vi "LockinEngine.Test.vi"(8 "error in (no error)":errorcluster, 11 "LockinDAQ in":refnum<class "LockinDAQ.lvclass">) -> (0 "error out":errorcluster, 3 "LockinDAQ out":refnum<class "LockinDAQ.lvclass">)   [LabVIEW 2016, in "LockinDAQ.lvclass"]
uses:
  LockinDAQ.lvclass
  Typedefs/Sampling.ctl
  <vilib>/Analysis/NI_AALBase.lvlib
  <vilib>/Analysis/baseanly.llb/Mean (DBL).vi
  Typedefs/AO_Amp-array.ctl
  Typedefs/AO_DC-array.ctl
  Typedefs/AO_phi-array.ctl
  Typedefs/Function-enum.ctl
  Typedefs/Function-array.ctl
  Typedefs/AO_f-array.ctl
  Typedefs/AO-cluster.ctl
  Typedefs/REF_f-array.ctl
  Typedefs/REF_phi-array.ctl
  Typedefs/REF-cluster.ctl
panel:
  out "Waveform Chart 2":u32(graph)
  out "Average time for each method (ms)":dbl[](array[numeric])
  in  "order":i32=2
  in  "TC (s)":dbl=0.3
  in  "Channels: Lockin":T1={"REF f (Hz)"=[13.0], "REF phi (°)"=[0.0]} {"REF phi (°)" format="%#_3g"}
  out "Waveform Chart":dbl[][](graph)
  in  "AO Chanels":T4={"AO Amp (V)"=[0.01], "AO DC (V)"=[0.0], "AO f (Hz)"=[13.0], "AO Phase (°)"=[0.0], "Function"=[enum."Sine"], "I+"=[], "Sweeping"=[FALSE]} {"AO f (Hz)" min=0.001 max=10000.0; "AO DC (V)" format="%.3p"; "AO Amp (V)" format="%.3p"}
  # "1"
  # "2"
  # "3"
  # "4"
  # "5"
  # "6"
  # "7"
  # "8"
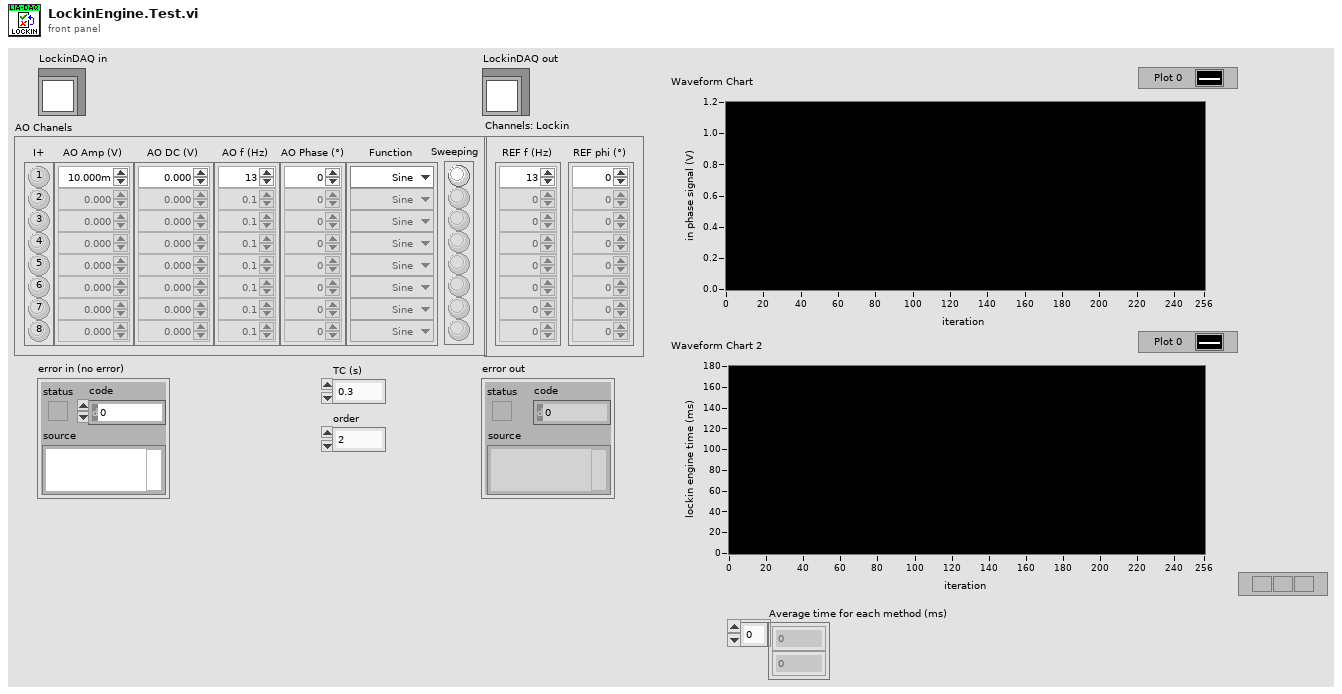
[diagram p1: front panel]
types:
  T1 = typedef "LockinDAQ.lvclass/REF-cluster.ctl" = cluster{"REF f (Hz)":T2, "REF phi (°)":T3}
  T2 = typedef "LockinDAQ.lvclass/REF_f-array.ctl" = dbl[]
  T3 = typedef "LockinDAQ.lvclass/REF_phi-array.ctl" = dbl[]
  T4 = typedef "LockinDAQ.lvclass/AO-cluster.ctl" = cluster{"AO Amp (V)":T5, "AO DC (V)":T6, "AO f (Hz)":T7, "AO Phase (°)":T8, "Function":T9, "I+":bool[], "Sweeping":bool[]}
  T5 = typedef "LockinDAQ.lvclass/AO_Amp-array.ctl" = dbl[]
  T6 = typedef "LockinDAQ.lvclass/AO_DC-array.ctl" = dbl[]
  T7 = typedef "LockinDAQ.lvclass/AO_f-array.ctl" = dbl[]
  T8 = typedef "LockinDAQ.lvclass/AO_phi-array.ctl" = dbl[]
  T9 = typedef "LockinDAQ.lvclass/Function-array.ctl" = T10[]
  T10 = typedef "LockinDAQ.lvclass/Function-enum.ctl" = enum16{"Sine", "Triangle", "Square", "Sawtooth"}
  T11 = enum16{"method 1", "method 2", "method 3", "method 4", "method 5"}[]
  T12 = typedef "LockinDAQ.lvclass/Sampling.ctl" = cluster{"Fs":dbl, "#s":i32}
  T13 = typedef "LockinDAQ.lvclass/Results--Cluster.ctl" = cluster{"Time Stamp":timestamp, "Results":dbl[][]}
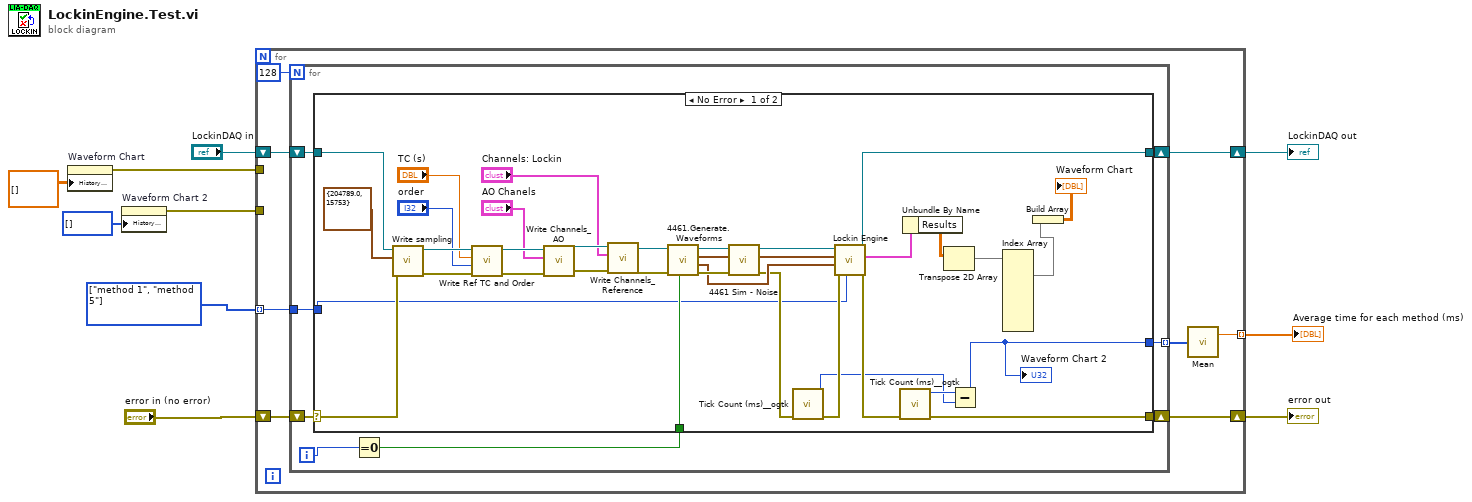
[diagram p0: block diagram]
diagram:
  w5 = T11 [enum."method 1", enum."method 5"] items=["method 1", "method 2", "method 3", "method 4", "method 5"]
  n1 = property on="Waveform Chart" class="WFChart (strict)"("History Data"=dbl[][] []) -> (error out=w3:errorcluster)  [unwired: 2 in, 1 out]
  n2 = property on="Waveform Chart 2" class="WFChart (strict)"("History Data"=u32[] []) -> (error out=w4:errorcluster)  [unwired: 2 in, 1 out]
  n3 = for {
    tunnel: [w11] -> w6 mode=indexing
    tunnel: w5 -> [w13] mode=indexing
    shift-right: [w17] -> w9
    shift-left: "error in (no error)" -> [w18]
    shift-right: [w15] -> w7
    shift-left: "LockinDAQ in" -> [w16]
    tunnel: w4 -> [_]
    tunnel: w3 -> [_]
    n4 = for {
      N: 128 -> [_]
      shift-right: [w25] -> w17
      shift-left: w18 -> [w26]
      shift-right: [w23] -> w15
      shift-left: w16 -> [w24]
      tunnel: [w22] -> w14 mode=indexing
      tunnel: w13 -> [w21]
      i -> [w20]
      n5 = Equal To 0?(x=w20) -> (x = 0?=w19:bool)
      n6 = case shown="No Error" w26 {
        selector: w26 -> [w57 w64]
        tunnel: [w35 w64] -> w25
        tunnel: [w52 w63] -> w23
        tunnel: w24 -> [w58 w63]
        tunnel: [w32 _] -> w22
        tunnel: w21 -> [w30 _]
        tunnel: w19 -> [w33 _]
        frame No Error {
          n7 = call "Write sampling.vi"("error in (no error)"=w57, "sampling"=T12 {"Fs"=204789.0, "#s"=15753}, "LockinDAQ"=w58) -> ("error out"=w45:errorcluster, "LockinDAQ out"=w46:refnum<class "LockinDAQ.lvclass">)  [unwired: 7 in]
          n8 = call "Write Ref TC and Order.vi"("error in (no error)"=w45, "order"="order", "TC (s)"="TC (s)", "LockinDAQ"=w46) -> ("error out"=w43:errorcluster, "LockinDAQ out"=w44:refnum<class "LockinDAQ.lvclass">)  [unwired: 6 in]
          n9 = call "Write Channels_ AO.vi"("error in (no error)"=w43, "Channels: AO"="AO Chanels", "LockinDAQ"=w44) -> ("error out"=w50:errorcluster, "LockinDAQ out"=w51:refnum<class "LockinDAQ.lvclass">)  [unwired: 7 in]
          n10 = call "Write Channels_ Reference.vi"("error in (no error)"=w50, "Channels: Lockin"="Channels: Lockin", "LockinDAQ"=w51) -> ("error out"=w48:errorcluster, "LockinDAQ out"=w49:refnum<class "LockinDAQ.lvclass">)  [unwired: 7 in]
          n11 = call "4461.Generate.Waveforms.vi"("Reset?"=w33, "error in (no error)"=w48, "LockinDAQ"=w49) -> ("error out"=w60:errorcluster, "REF []"=w38:waveform(dbl)[], "AO []"=w62:waveform(dbl)[], "LockinDAQ out"=w61:refnum<class "LockinDAQ.lvclass">)  [unwired: 5 in]
          n12 = call "4461 Sim - Noise.vi"("error in (no error)"=w60, "AO []"=w62, "LockinDAQ"=w61) -> ("error out"=w37:errorcluster, "\"AI\" []"=w56:waveform(dbl)[], "LockinDAQ out"=w55:refnum<class "LockinDAQ.lvclass">)  [unwired: 6 in]
          n13 = call <userlib>:"Tick Count (ms)__ogtk.vi"("error in (no error)"=w37) -> ("error out"=w36:errorcluster, "millisecond timer value"=w29:u32)  [unwired: 9 in]
          n14 = call "Lockin Engine.vi"(6:w30, "error in (no error)"=w36, "Reference In"=w38, "Signal in"=w56, "LockinDAQ"=w55) -> ("error out"=w31:errorcluster, "Results (X,Y,R,Theta,Mean)"=w39:T13, "LockinDAQ out"=w52:refnum<class "LockinDAQ.lvclass">)  [unwired: 3 in, 1 out]
          n15 = call <userlib>:"Tick Count (ms)__ogtk.vi"("error in (no error)"=w31) -> ("error out"=w35:errorcluster, "millisecond timer value"=w34:u32)  [unwired: 9 in]
          n16 = Unbundle By Name(w39) -> ("Results"=w53:dbl[][])
          n17 = Transpose 2D Array(2D array=w53) -> (transposed array=w54:dbl[][])
          n18 = Subtract(x=w34, y=w29) -> (x-y=w32:u32)
          "Waveform Chart 2" <- w32
          n19 = Index Array(array=w54) -> (element #1=w28:dbl[])  [unwired: 8 in, 3 out]
          n20 = Build Array(w28) -> (→"Waveform Chart":dbl[][])
        }
        frame Error {
        }
      }
    }
    n21 = call-poly <vilib>:"Mean.vi"("X"=w14) -> ("mean"=w11:dbl)  [unwired: 1 out]
  }
  "error out" <- w9
  "LockinDAQ out" <- w7
  "Average time for each method (ms)" <- w6
